vi "FPGA_Main.vi"() -> ()   [LabVIEW 2018]
uses:
  <vilib>/rvi/FXPMathLib/FxpDiv/subVIs/nifxpmath_Div_SimConfig.ctl
  <vilib>/rvi/FXPMathLib/FxpAtan2/subVIs/nifxpmath_Atan2_SimConfig.ctl
  <vilib>/rvi/FXPMathLib/FxpSinAndCos/subVIs/nifxpmath_SinAndCos_SimConfig.ctl
  <vilib>/rvi/Emulation/niFpgaGetClockAttributes.vi
  <vilib>/rvi/Emulation/niFpgaSctlEmulationGetInTimedLoop.vi
  <vilib>/rvi/Emulation/niFpgaEmulationReportErrorSimple.vi
  <vilib>/rvi/eio/common/nirviEmuTemplateMethod_errors.vi
  <vilib>/rvi/Emulation/niFpgaProcessEmulError.vi
  <vilib>/rvi/FXPMathLib/FxpDiv/simVIs/DllFxpDivTemp_sub.vi
  <vilib>/rvi/FXPMathLib/FxpAtan2/simVIs/DllFxpAtan2Temp_sub.vi
  <vilib>/rvi/FXPMathLib/FxpSinAndCos/simVIs/DllFxpSinAndCosTemp_sub.vi
  <vilib>/rvi/interface/RandomDataEmulation/nirviRandomDataMultiElementFPGAFIFO.vi
  <instcachedir>/0/nirviRandomDataMultiElementFPGAFIFO_6740B454F3C245F78F76ED91F73FD8DB.lvgen/nirviRandomDataMultiElementFPGAFIFO_6740B454F3C245F78F76ED91F73FD8DB_007.vi
  <vilib>/rvi/interface/RandomDataEmulation/niFpgaRandomDataHandleErrors.vi
  <vilib>/rvi/Emulation/niFpgaCriticalErrorInLSC.vi
  <vilib>/eio/EIONode/EIONode.xnode
  <vilib>/rvi/FXPMathLib/FxpMul/XNode/nifxpmath_Multiplier.xnode
  <vilib>/rvi/Analysis/measure/butterworth/XNode/niFpgaButterworthFilter.xnode
  <vilib>/rvi/FXPMathLib/FxpSub/XNode/nifxpmath_Sub.xnode
  <vilib>/rvi/FXPMathLib/FxpDiv/XNode/nifxpmath_Div.xnode
  <vilib>/rvi/Analysis/measure/notch/XNode/niFpgaNotchFilter.xnode
  <vilib>/rvi/FXPMathLib/FxpAtan2/XNode/nifxpmath_Atan2.xnode
  <vilib>/rvi/FXPMathLib/FxpAdd/XNode/nifxpmath_Add.xnode
  <vilib>/rvi/FXPMathLib/FxpSinAndCos/XNode/nifxpmath_SinAndCos.xnode
  <vilib>/rvi/DataTransferAndStorage/Container/XNode/niFpgaContainer.xnode
  <vilib>/rvi/interface/RandomDataEmulation/nirviRandomDataFpgaMultiElementTemplate.vi
  <vilib>/rvi/FXPMathLib/sim/FxpSim.dll
panel:
  in  "phase_correction":fxp<+/-,16,2>[](array[numeric])=[0.0, 0.0, 0.0]
  in  "idx scope":u8=25
  in  "gain":fxp<+,18,6>=1.0
  in  "base freqs":fxp<+,17,17>[](array[numeric])=[0.0, 0.0, 0.0]
  in  "idx pick":u8=25
  in  "reset":bool
  in  "I gain":fxp<+,20,6>
  in  "P gain":fxp<+,14,14>=700.0
  # "FPGA Main"
  # "Shared variables for interaction with RT- and PC-Main"
  # "Enable only in simulation mode!"
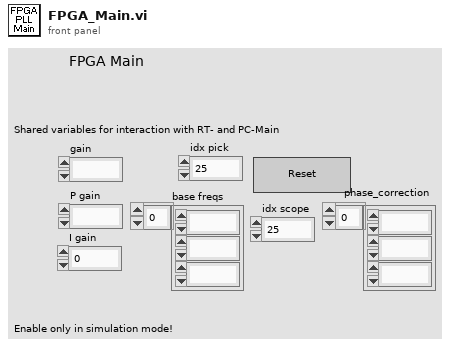
[diagram p1: front panel]
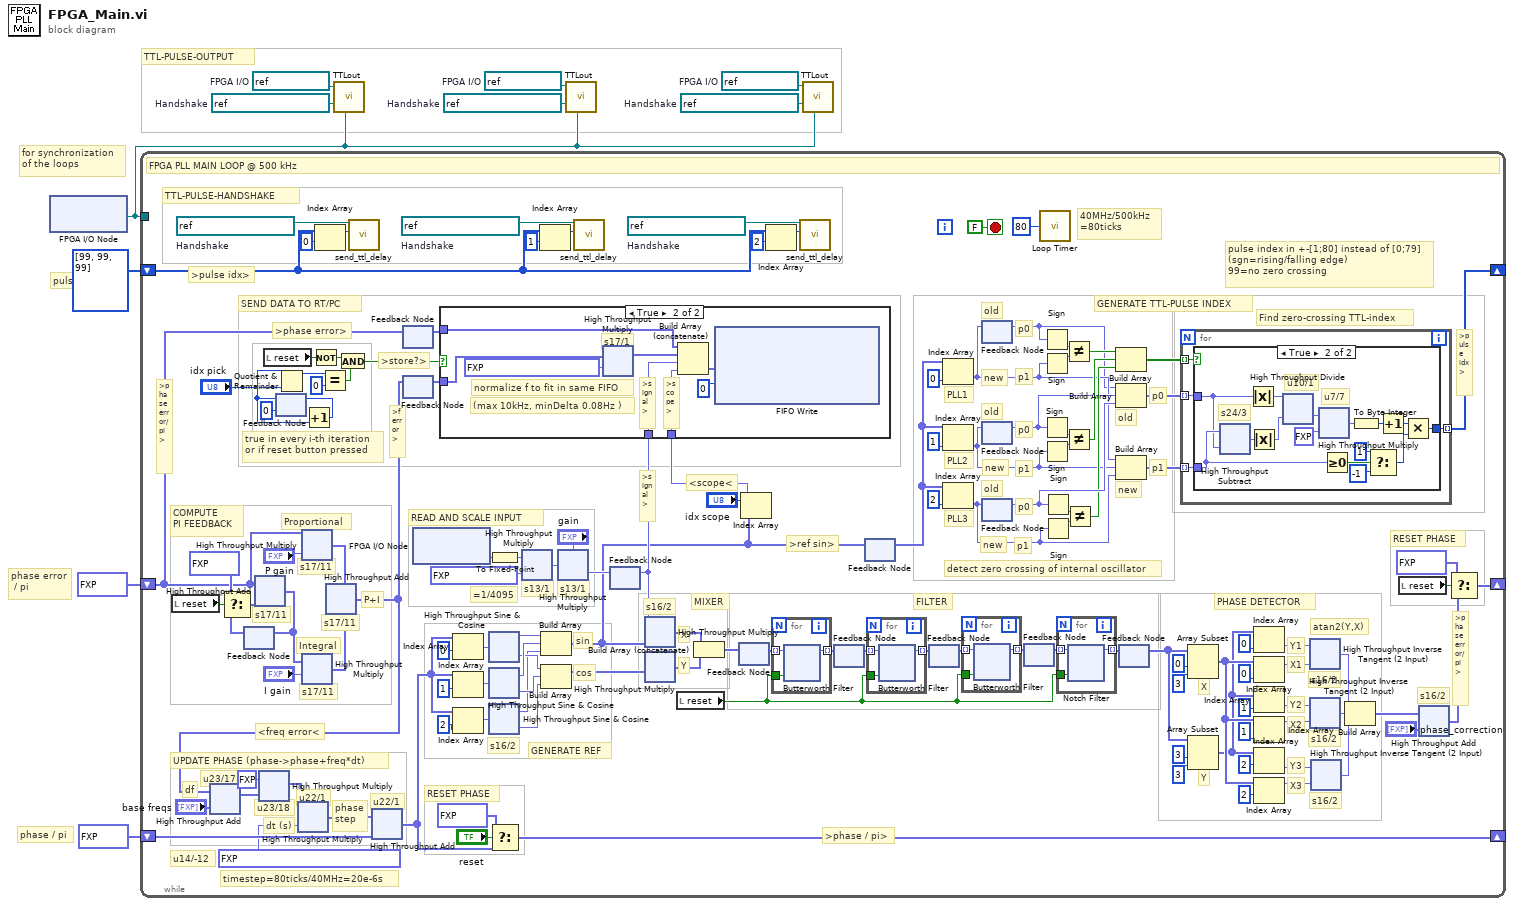
[diagram p0: block diagram]
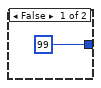
[diagram p2: hidden frame]
diagram:
  w3 = refnum<k21> "TTL-out3"  # FPGA I/O
  w2 = refnum<k21> "TTL_Handshake3"  # Handshake
  w4 = refnum<k21> "TTL-out2"  # FPGA I/O
  w5 = refnum<k21> "TTL_Handshake2"  # Handshake
  w7 = refnum<k21> "TTL-out1"  # FPGA I/O
  w6 = refnum<k21> "TTL_Handshake1"  # Handshake
  # "TTL-PULSE-OUTPUT"
  # "for synchronization\nof the loops"
  # "pulse idx"
  # "phase error\n / pi"
  # "phase / pi"
  n1 = xnode "FPGA I/O Node"() -> ("FPGA I/O Out"=w1:refnum<k21>)  [unwired: 1 in, 1 out]
  n2 = while {
    shift-right: [w142] -> _
    shift-left: fxp<+/-,1,0>[] [0.0, 0.0, 0.0] ("t") -> [w141]
    shift-right: [w140] -> _
    shift-left: fxp<+/-,16,2>[] [0.0, 0.0, 0.0] ("t") -> [w83]
    shift-right: [w50] -> _
    shift-left: i8[] [99, 99, 99] ("idx array") -> [w77]
    tunnel: w1 -> [_]
    stop <- FALSE stop-if-true
    w80 = refnum<k21> "TTL_Handshake3"  # Handshake
    w133 = refnum<k21> "TTL_Handshake2"  # Handshake
    w138 = refnum<k21> "TTL_Handshake1"  # Handshake
    # "s16/2"
    # ">phase error/pi>"
    # "Y"
    # "X"
    # "FILTER"
    # "MIXER"
    # "<scope<"
    # ">pulse idx>"
    # ">pulse idx>"
    # ">store?>"
    # ">phase error>"
    # ">signal>"
    # "s16/2"
    # "X3"
    # "Y3"
    # "X2"
    # "Y2"
    # "X1"
    # "Y1"
    # "40MHz/500kHz\n=80ticks"
    # "COMPUTE\nPI FEEDBACK"
    # "GENERATE TTL-PULSE INDEX"
    # "pulse index in +-[1;80] instead of [0;79]\n(sgn=rising/falling edge)\n99=no zero crossing"
    # "Find zero-crossing TTL-index"
    # "detect zero crossing of internal oscillator"
    # "s16/2"
    # "PHASE DETECTOR"
    # ">ref sin>"
    # "new"
    # "old"
    # "PLL3"
    # "p1"
    # "p0"
    # "new"
    # "old"
    # "p1"
    # "p0"
    # "PLL2"
    # "PLL1"
    # "p1"
    # "p0"
    # "new"
    # "old"
    # "p1"
    # "p0"
    # "new"
    # "old"
    # "s16/2"
    # "s16/2"
    # "atan2(Y,X)"
    # "dt (s)"
    # "u23/17"
    # "u23/18"
    # "u22/1"
    # "u22/1"
    # "df"
    # "UPDATE PHASE (phase->phase+freq*dt)"
    # "phase\nstep"
    # "s17/11"
    # "s17/11"
    # "s17/11"
    # "s17/11"
    # "P+I"
    # "Integral"
    # "Proportional"
    # "u14/-12"
    # "timestep=80ticks/40MHz=20e-6s"
    # "Y"
    # "X"
    # "s13/1"
    # "READ AND SCALE INPUT"
    # "true in every i-th iteration \nor if reset button pressed"
    # "SEND DATA TO RT/PC"
    # ">phase error/pi>"
    # "GENERATE REF"
    # "cos"
    # "sin"
    # "<freq error<"
    # "s16/2"
    # "s13/1"
    # "=1/4095"
    # "RESET PHASE"
    # ">f error>"
    # "RESET PHASE"
    # ">phase / pi>"
    # "TTL-PULSE-HANDSHAKE"
    # "FPGA PLL MAIN LOOP @ 500 kHz"
    n3 = local read "reset"() -> (w93:bool)
    n4 = feedback #1() -> (w94:fxp<+/-,17,11>[])  [unwired: 1 in]
    n5 = Select(t=fxp<+/-,16,10>[] [0.0, 0.0, 0.0], s=w93, f=w94) -> (s? t:f=w82:fxp<+/-,17,11>[])
    n6 = xnode ("High Throughput Add")("x"=w83, "y"=w82) -> ("x+y"=w84:fxp<+/-,17,11>[])
    n7 = feedback-in #1(w84) -> ()
    n8 = local read "reset"() -> (w124:bool)
    n9 = feedback #2(i16 0) -> (w123:i16)
    n10 = Quotient & Remainder(x=w123, y="idx pick") -> (x-y*floor(x/y)=w129:i16)  [unwired: 1 out]
    n11 = xnode ("High Throughput Multiply")("x"=w83, "y"="P gain") -> ("x*y"=w97:fxp<+/-,17,11>[])
    n12 = xnode ("High Throughput Multiply")("x"=w84, "y"="I gain") -> ("x*y"=w98:fxp<+/-,17,11>[])
    n13 = Increment(x=w123) -> (x+1=w122:i16)
    n14 = feedback-in #2(w122) -> ()
    n15 = Not(x=w124) -> (.not. x?=w125:bool)
    n16 = Index Array(array=w77, index=0) -> (element=w136:i8)
    n17 = Equal?(x=w129, y=i16 0) -> (x = y?=w121:bool)
    n18 = xnode ("High Throughput Add")("x"=w97, "y"=w98) -> ("x+y"=w32:fxp<+/-,17,11>[])
    n19 = xnode ("High Throughput Add")("x"=w32, "y"="base freqs") -> ("x+y"=w89:fxp<+,23,17>[])
    n20 = xnode ("High Throughput Multiply")("x"=fxp<+,2,2> 2.0 ("y"), "y"=w89) -> ("x*y"=w91:fxp<+,23,18>[])
    n21 = xnode ("High Throughput Multiply")("x"=w91, "y"=fxp<+,14,-18> 2.00001522898674e-06) -> ("x*y"=w90:fxp<+,22,1>[])
    n22 = And(x=w125, y=w121) -> (x .and. y?=w126:bool)
    n23 = call "send_ttl_delay.vi"("delay index"=w136, "Handshake"=w138) -> ()  [unwired: 10 in]
    n24 = xnode ("High Throughput Add")("x"=w90, "y"=w141) -> ("x+y"=w51:fxp<+,22,1>[])
    n25 = feedback #3() -> (w107:fxp<+/-,16,2>[])  [unwired: 1 in]
    n26 = feedback-in #3(w83) -> ()
    n27 = feedback #4() -> (w108:fxp<+/-,17,11>[])  [unwired: 1 in]
    n28 = feedback-in #4(w32) -> ()
    n29 = xnode "FPGA I/O Node"() -> ("REF-in"=w106:i16)  [unwired: 1 in, 1 out]
    n30 = Index Array(array=w51, index=0) -> (element=w115:fxp<+,22,1>)
    n31 = Index Array(array=w51, index=1) -> (element=w114:fxp<+,22,1>)
    n32 = Index Array(array=w51, index=2) -> (element=w76:fxp<+,22,1>)
    n33 = xnode "High Throughput Sine & Cosine"("x (pi)"=w115) -> ("sin(x)"=w113:fxp<+/-,16,2>, "cos(x)"=w111:fxp<+/-,16,2>)
    n34 = xnode "High Throughput Sine & Cosine"("x (pi)"=w114) -> ("sin(x)"=w112:fxp<+/-,16,2>, "cos(x)"=w110:fxp<+/-,16,2>)
    n35 = xnode "High Throughput Sine & Cosine"("x (pi)"=w76) -> ("sin(x)"=w73:fxp<+/-,16,2>, "cos(x)"=w74:fxp<+/-,16,2>)
    n36 = To Fixed-Point(number=w106) -> (fixed-point=w132:fxp<+/-,12,12>)  [unwired: 1 in]
    n37 = Select(t=fxp<+/-,1,0>[] [0.0, 0.0, 0.0], s="reset", f=w51) -> (s? t:f=w142:fxp<+/-,23,2>[])
    n38 = xnode ("High Throughput Multiply")("x"=w132, "y"=fxp<+,12,0> 0.000244140625) -> ("x*y"=w102:fxp<+/-,13,1>)
    n39 = Index Array(array=w77, index=1) -> (element=w135:i8)
    n40 = Build Array(w113, w112, w73) -> (w15:fxp<+/-,16,2>[])
    n41 = Build Array(w111, w110, w74) -> (w109:fxp<+/-,16,2>[])
    n42 = xnode ("High Throughput Multiply")("x"="gain", "y"=w102) -> ("x*y"=w101:fxp<+/-,13,1>)
    n43 = call "send_ttl_delay.vi"("delay index"=w135, "Handshake"=w133) -> ()  [unwired: 10 in]
    n44 = feedback #5() -> (w105:fxp<+/-,13,1>)  [unwired: 1 in]
    n45 = feedback-in #5(w101) -> ()
    n46 = xnode ("High Throughput Multiply")("x"=w105, "y"=w15) -> ("x*y"=w41:fxp<+/-,16,2>[])
    n47 = xnode ("High Throughput Multiply")("x"=w105, "y"=w109) -> ("x*y"=w40:fxp<+/-,16,2>[])
    n48 = local read "reset"() -> (w19:bool)
    n49 = Build Array (concatenate)(w41, w40) -> (w39:fxp<+/-,16,2>[])
    n50 = feedback #6() -> (w16:fxp<+/-,16,2>[])  [unwired: 1 in]
    n51 = feedback-in #6(w39) -> ()
    n52 = Index Array(array=w15, index="idx scope") -> (element=w48:fxp<+/-,16,2>)
    n53 = case shown="True" w126 {
      tunnel: w107 -> [_ w415]
      tunnel: w105 -> [_ w414]
      tunnel: w108 -> [_ w413]
      tunnel: w48 -> [_ w412]
      frame False {
      }
      frame True {
        # ">scope>"
        # "(max 10kHz, minDelta 0.08Hz )"
        # ">signal>"
        # "normalize f to fit in same FIFO"
        # "s17/1"
        # "send data until queue is full"
        n54 = xnode ("High Throughput Multiply")("x"=w413, "y"=fxp<+/-,22,1> 0.00010013580322265625) -> ("x*y"=w416:fxp<+/-,17,1>[])
        n55 = Build Array (concatenate)(w415, w416, w414, w412) -> (w417:fxp<+/-,18,2>[])
        n56 = xnode ("FIFO Write")("Element"=w417, "Timeout"=i16 0) -> ()  [unwired: 1 in, 2 out]
      }
    }
    n57 = Index Array(array=w77, index=2) -> (element=w78:i8)
    n58 = for {
      tunnel: w19 -> [w181]
      tunnel: w16 -> [w180] mode=indexing
      tunnel: [w179] -> w24 mode=indexing
      n59 = xnode "Butterworth Filter"("input data"=w180, "reset"=w181) -> ("output data"=w179:fxp<+/-,16,2>)  [unwired: 1 in, 1 out]
    }
    n60 = call "send_ttl_delay.vi"("delay index"=w78, "Handshake"=w80) -> ()  [unwired: 10 in]
    n61 = feedback #7() -> (w25:fxp<+/-,16,2>[])  [unwired: 1 in]
    n62 = feedback-in #7(w24) -> ()
    n63 = feedback #8() -> (w14:fxp<+/-,16,2>[])  [unwired: 1 in]
    n64 = feedback-in #8(w15) -> ()
    n65 = for {
      tunnel: w19 -> [w169]
      tunnel: w25 -> [w168] mode=indexing
      tunnel: [w167] -> w20 mode=indexing
      n66 = xnode "Butterworth Filter"("input data"=w168, "reset"=w169) -> ("output data"=w167:fxp<+/-,16,2>)  [unwired: 1 in, 1 out]
    }
    n67 = feedback #9() -> (w21:fxp<+/-,16,2>[])  [unwired: 1 in]
    n68 = feedback-in #9(w20) -> ()
    n69 = Index Array(array=w14, index=0) -> (element=w61:fxp<+/-,16,2>)
    n70 = Index Array(array=w14, index=1) -> (element=w66:fxp<+/-,16,2>)
    n71 = Index Array(array=w14, index=2) -> (element=w71:fxp<+/-,16,2>)
    n72 = for {
      tunnel: w19 -> [w155]
      tunnel: w21 -> [w157] mode=indexing
      tunnel: [w156] -> w22 mode=indexing
      n73 = xnode "Butterworth Filter"("input data"=w157, "reset"=w155) -> ("output data"=w156:fxp<+/-,16,2>)  [unwired: 1 in, 1 out]
    }
    n74 = feedback #10() -> (w60:fxp<+/-,16,2>)  [unwired: 1 in]
    n75 = feedback-in #10(w61) -> ()
    n76 = feedback #11() -> (w65:fxp<+/-,16,2>)  [unwired: 1 in]
    n77 = feedback-in #11(w66) -> ()
    n78 = feedback #12() -> (w72:fxp<+/-,16,2>)  [unwired: 1 in]
    n79 = feedback-in #12(w71) -> ()
    n80 = feedback #13() -> (w23:fxp<+/-,16,2>[])  [unwired: 1 in]
    n81 = feedback-in #13(w22) -> ()
    n82 = call "Loop Timer"("Count(Ticks)"=u32 80) -> ()  [unwired: 1 out]
    n83 = Sign(1:w60) -> (0:w58:fxp<+/-,2,2>)
    n84 = Sign(1:w61) -> (0:w59:fxp<+/-,2,2>)
    n85 = Sign(1:w65) -> (0:w64:fxp<+/-,2,2>)
    n86 = Sign(1:w66) -> (0:w63:fxp<+/-,2,2>)
    n87 = Sign(1:w72) -> (0:w68:fxp<+/-,2,2>)
    n88 = Sign(1:w71) -> (0:w69:fxp<+/-,2,2>)
    n89 = for {
      tunnel: w19 -> [w143]
      tunnel: w23 -> [w145] mode=indexing
      tunnel: [w144] -> w18 mode=indexing
      n90 = xnode "Notch Filter"("input data"=w145, "reset"=w143) -> ("output data"=w144:fxp<+/-,16,2>)  [unwired: 1 in, 1 out]
    }
    n91 = Not Equal?(x=w58, y=w59) -> (x != y?=w62:bool)
    n92 = Not Equal?(x=w64, y=w63) -> (x != y?=w67:bool)
    n93 = Not Equal?(x=w68, y=w69) -> (x != y?=w70:bool)
    n94 = Build Array(w62, w67, w70) -> (w56:bool[])
    n95 = Build Array(w60, w65, w72) -> (w55:fxp<+/-,16,2>[])
    n96 = Build Array(w61, w66, w71) -> (w57:fxp<+/-,16,2>[])
    n97 = feedback #14() -> (w17:fxp<+/-,16,2>[])  [unwired: 1 in]
    n98 = feedback-in #14(w18) -> ()
    n99 = for {
      tunnel: w55 -> [w194] mode=indexing
      tunnel: w56 -> [w193] mode=indexing
      tunnel: w57 -> [w192] mode=indexing
      tunnel: [w191] -> w50 mode=indexing
      n100 = case shown="True" w193 {
        tunnel: w194 -> [_ w196]
        tunnel: w192 -> [_ w204]
        tunnel: [i8 99 w206] -> w191
        frame False {
        }
        frame True {
          # "u7/7"
          # "u10/1"
          # "s24/3"
          n101 = xnode "High Throughput Subtract"("x"=w204, "y"=w196) -> ("x-y"=w199:fxp<+/-,24,3>)
          n102 = Absolute Value(x=w196) -> (abs(x)=w197:fxp<+,16,2>)
          n103 = Absolute Value(x=w199) -> (abs(x)=w198:fxp<+,24,3>)
          n104 = xnode "High Throughput Divide"("x"=w197, "y"=w198) -> ("x/y"=w209:fxp<+,10,1>)
          n105 = xnode ("High Throughput Multiply")("x"=w209, "y"=fxp<+,7,7> 79.0 ("x")) -> ("x*y"=w210:fxp<+,7,7>)
          n106 = Greater Or Equal To 0?(x=w204) -> (x >= 0?=w205:bool)
          n107 = To Byte Integer(number=w210) -> (8bit integer=w200:i8)
          n108 = Select(t=i8 1 ("index"), s=w205, f=i8 -1 ("index")) -> (s? t:f=w201:i8)
          n109 = Increment(x=w200) -> (x+1=w207:i8)
          n110 = Multiply(x=w207, y=w201) -> (x*y=w206:i8)
        }
      }
    }
    n111 = Array Subset(array=w17, index=0 ("length"), length=3) -> (w34:fxp<+/-,16,2>[])
    n112 = Array Subset(array=w17, index=3 ("length"), length=3) -> (w33:fxp<+/-,16,2>[])
    n113 = Index Array(array=w33, index=0) -> (element=w31:fxp<+/-,16,2>)
    n114 = Index Array(array=w34, index=0) -> (element=w30:fxp<+/-,16,2>)
    n115 = Index Array(array=w33, index=1) -> (element=w29:fxp<+/-,16,2>)
    n116 = Index Array(array=w34, index=1) -> (element=w28:fxp<+/-,16,2>)
    n117 = Index Array(array=w33, index=2) -> (element=w27:fxp<+/-,16,2>)
    n118 = Index Array(array=w34, index=2) -> (element=w26:fxp<+/-,16,2>)
    n119 = xnode "High Throughput Inverse Tangent (2 Input)"("y"=w31, "x"=w30) -> ("atan2(y,x) (pi)"=w86:fxp<+/-,16,2>)
    n120 = xnode "High Throughput Inverse Tangent (2 Input)"("y"=w29, "x"=w28) -> ("atan2(y,x) (pi)"=w87:fxp<+/-,16,2>)
    n121 = xnode "High Throughput Inverse Tangent (2 Input)"("y"=w27, "x"=w26) -> ("atan2(y,x) (pi)"=w81:fxp<+/-,16,2>)
    n122 = Build Array(w86, w87, w81) -> (w12:fxp<+/-,16,2>[])
    n123 = local read "reset"() -> (w130:bool)
    n124 = xnode ("High Throughput Add")("x"=w12, "y"="phase_correction") -> ("x+y"=w11:fxp<+/-,16,2>[])
    n125 = Select(t=fxp<+/-,1,0>[] [0.0, 0.0, 0.0], s=w130, f=w11) -> (s? t:f=w140:fxp<+/-,16,2>[])
  }
  n126 = call "TTLout.vi"("synch_signal"=w1, "Handshake"=w6, "FPGA I/O"=w7) -> ()  [unwired: 9 in]
  n127 = call "TTLout.vi"("synch_signal"=w1, "Handshake"=w5, "FPGA I/O"=w4) -> ()  [unwired: 9 in]
  n128 = call "TTLout.vi"("synch_signal"=w1, "Handshake"=w2, "FPGA I/O"=w3) -> ()  [unwired: 9 in]
